vi "make arbitrary waveform_grMD.vi"() -> ()   [LabVIEW 2017]
doc: "SciScan 1.2 160622"
uses:
  Custom Controls/scan mode main settings tab.ctl
  Custom Controls/pixel resolution enum.ctl
  Custom Controls/experiment type.ctl
  GFG/GFGDisplayRefsGet.vi
  GFG/GFGnumericGet.vi
  GFG/GFGfpRefGet.vi
  GFG/GFGImageRefsGet.vi
  GFG/GFGpathGet.vi
  GFG/GFG library.lvlib
  <vilib>/vision/NI_Vision_Development_Module.lvlib
panel:
  out "error out 5":errorcluster
  out "error out 4":errorcluster
  out "XY voltages of the current framescan":dbl[][][](array[numeric])
  out "x.pixels refreshed?":bool
  out "xy.voltage.map refreshed?":bool
  out "Linescan voltages refreshed?":bool
  out "linescan.xy.waveform refreshed?":bool
  out "ROI refreshed?":bool
  out "Source VI":string
  out "error out 3":errorcluster
  out "error out 2":errorcluster
  out "error out":errorcluster
  out "XY map":cluster{"Y":dbl[], "Y":dbl[]}[](graph)
  out "Final linescan xy voltage plot":cluster{"Y":dbl[], "Y":dbl[]}[](graph)
  out "XY linescan pixel map":cluster{"Y":dbl[], "Y":dbl[]}[](graph)
  out "Linescan y voltages per scan point":dbl[](graph)
  out "Linescan x voltages per scan point":dbl[](graph)
  out "Linescan y waveform":waveform(dbl)(graph)
  out "Linescan x waveform":waveform(dbl)(graph)
  out "Number of pixels per period":i32
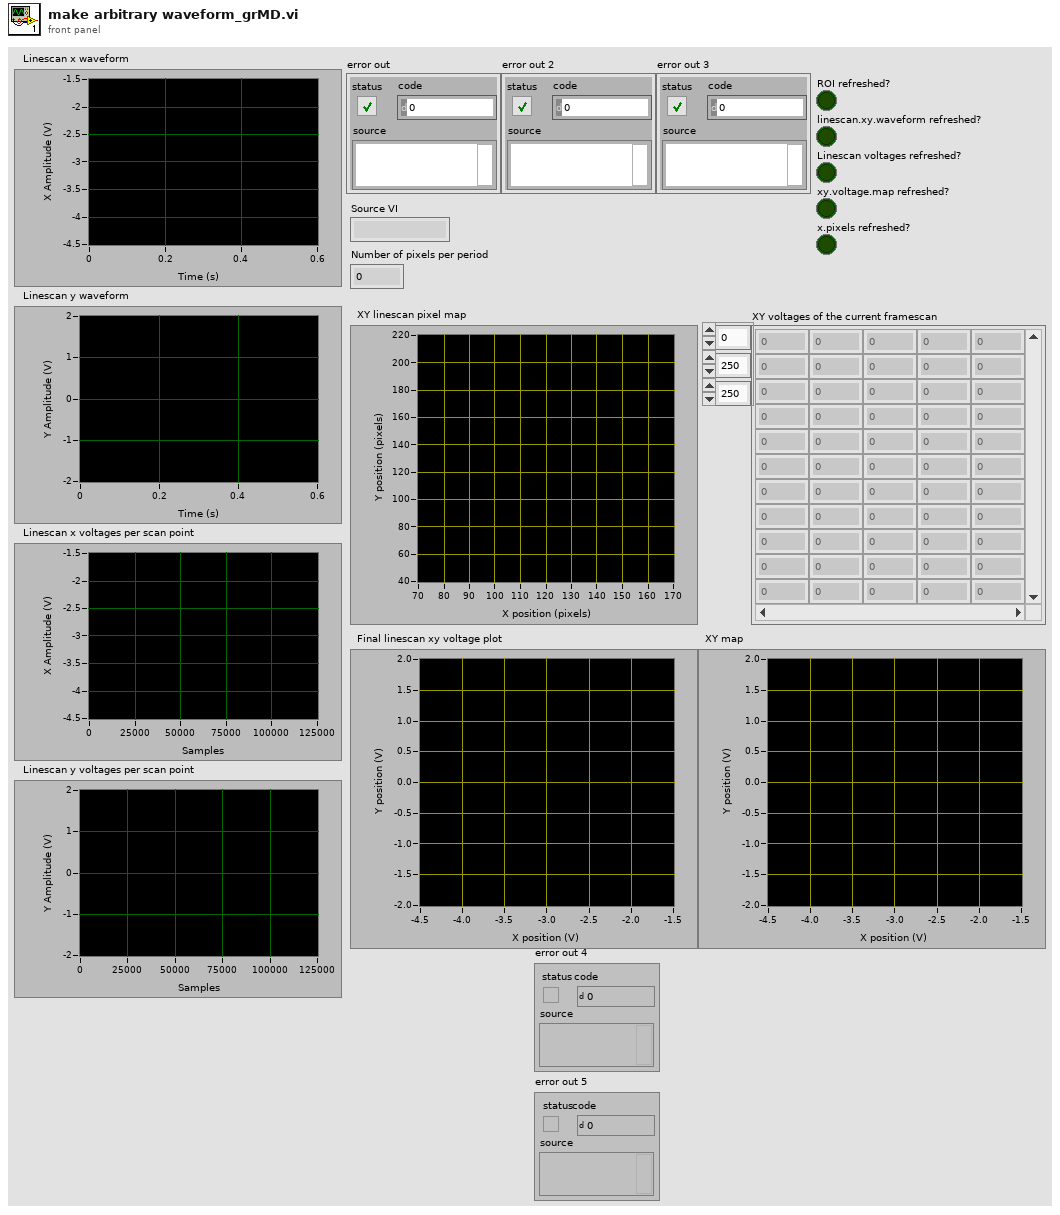
[diagram p1: front panel]
types:
  T1 = typedef "ROI Descriptor" = cluster{"Global Rectangle":i32[], "Contours":cluster{"ID":enum32{"External", "Internal"}, "Type":u32, "Coordinates":i32[]}[]}
  T2 = cluster{"Channel 1 small":refnum<vi>, "Channel 2 small":refnum<vi>, "Channel 3 small":refnum<vi>, "Channel 4 small":refnum<vi>, "Channel 1 large":refnum<vi>, "Channel 2 large":refnum<vi>, "Channel 3 large":refnum<vi>, "Channel 4 large":refnum<vi>, "RGB overlay":refnum<vi>, "ROI Image display":refnum<vi>, "arb line scan display":refnum<vi>, "Channel 5 large":refnum<vi>}
  T3 = cluster{"Global Rectangle":i32[], "Contours":cluster{"Contour Type":u32, "ROI Type":u32, "Points":i32[]}[]}
  T4 = cluster{"xyvoltagefor2frames":dbl[][][], "x.pixels":dbl, "nomin.x.pixels":dbl, "y.pixels":dbl, "fill.fraction":dbl, "x.bidirectional":bool, "y.bidirectional":bool}
  T5 = enum32{"Page Enabled", "Page Disabled", "Page Disabled & Grayed"}
  T6 = typedef "pixel resolution enum.ctl" = enum16{"128 x 128", "256 x 128", "256 x 256", "512 x  64", "512 x 128", "512 x 256", "512 x 512", "1024 x 512", "1024 x 1024", "arbitrary"}
  T7 = typedef "experiment type.ctl" = string
  T8 = enum8{"Enabled", "Disabled", "Disabled and Grayed Out"}
  T9 = typedef "scan mode main settings tab.ctl" = enum32{"2D frame", "2D line scan", "general settings", "Z Stack", "piezo"}
  T10 = cluster{"WaveformChartRef":refnum<vi>, "DigitalRef":refnum<vi>, "ArrayRef":refnum<vi>, "TabControlRef":refnum<vi>, "EnumRef":refnum<vi>, "RingRef":refnum<vi>, "BooleanRef":refnum<vi>, "KnobRef":refnum<vi>, "SlideRef":refnum<vi>, "PathRef":refnum<vi>, "StringRef":refnum<vi>, "ComboBox":refnum<vi>, "WaveformGraphRef":refnum<vi>}
  T11 = typedef "IMAQ Image.ctl" = refnum<image>
  T12 = cluster{"Channel 1 small":T11, "Channel 2 small":T11, "Channel 3 small":T11, "Channel 4 small":T11, "Channel 1 large":T11, "Channel 2 large":T11, "Channel 3 large":T11, "Channel 4 large":T11, "RGB overlay":T11, "ROI Image display":T11, "arb line scan display":T11, "Channel 5 large":T11}
  T13 = cluster{"ID":enum32{"External", "Internal"}, "Type":u32, "Coordinates":i32[]}[]
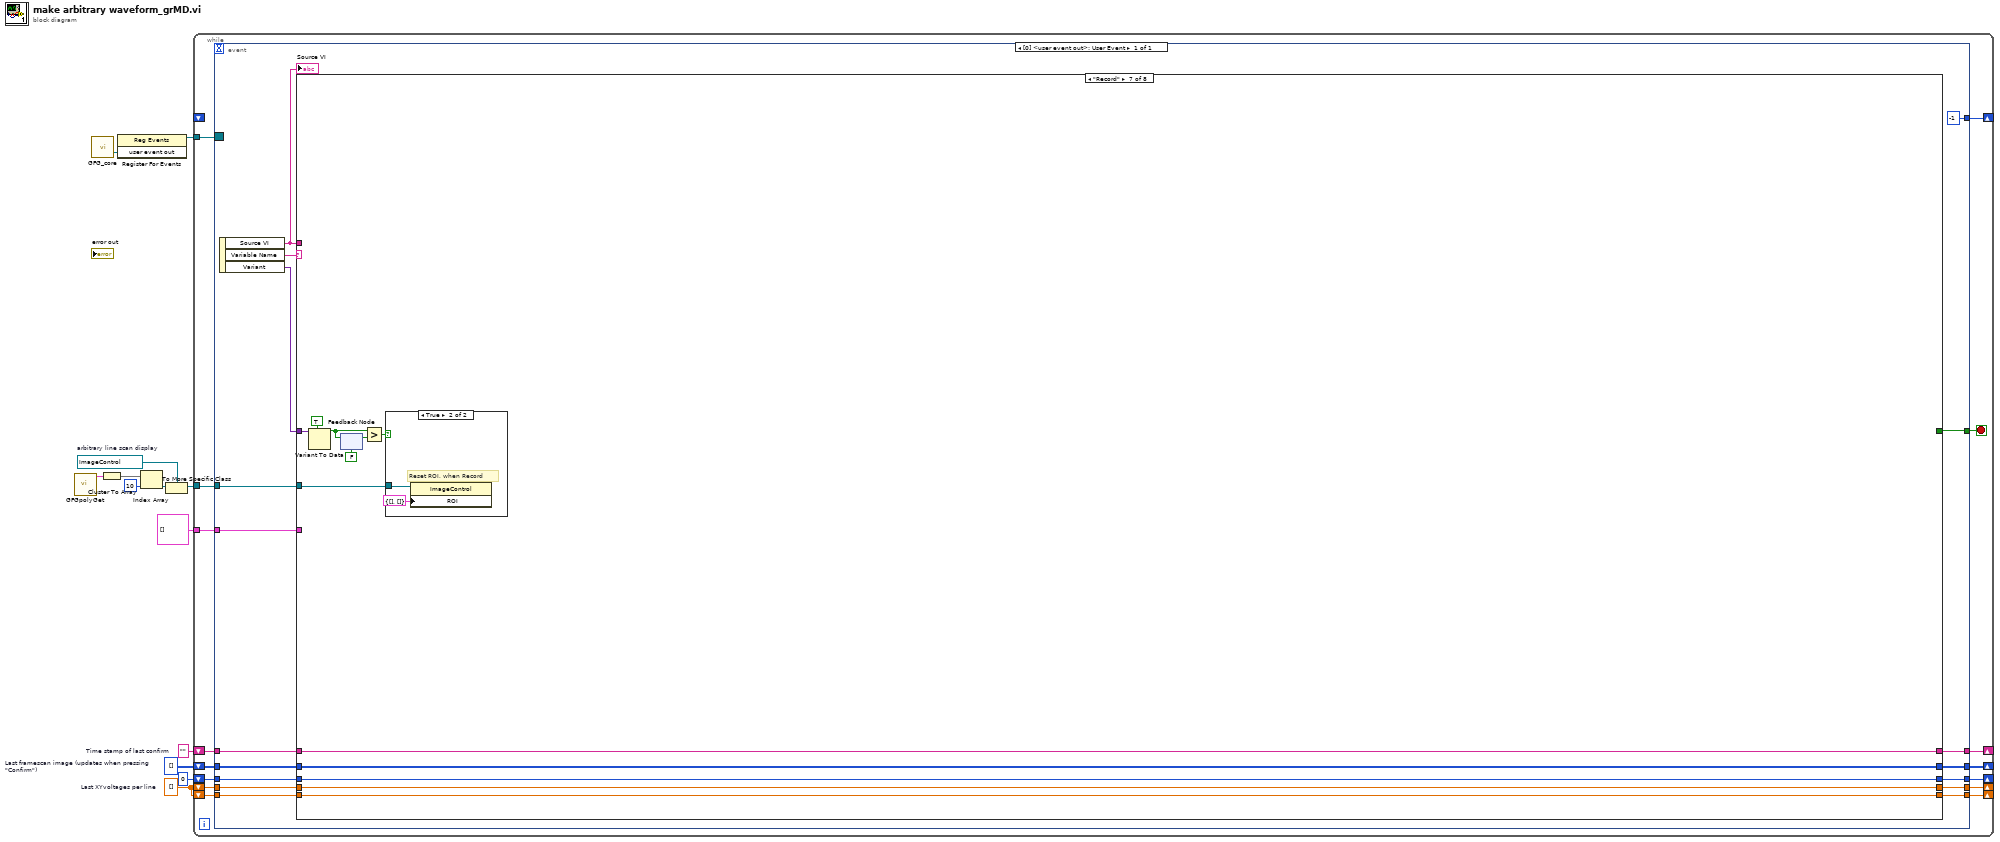
[diagram p0: block diagram]
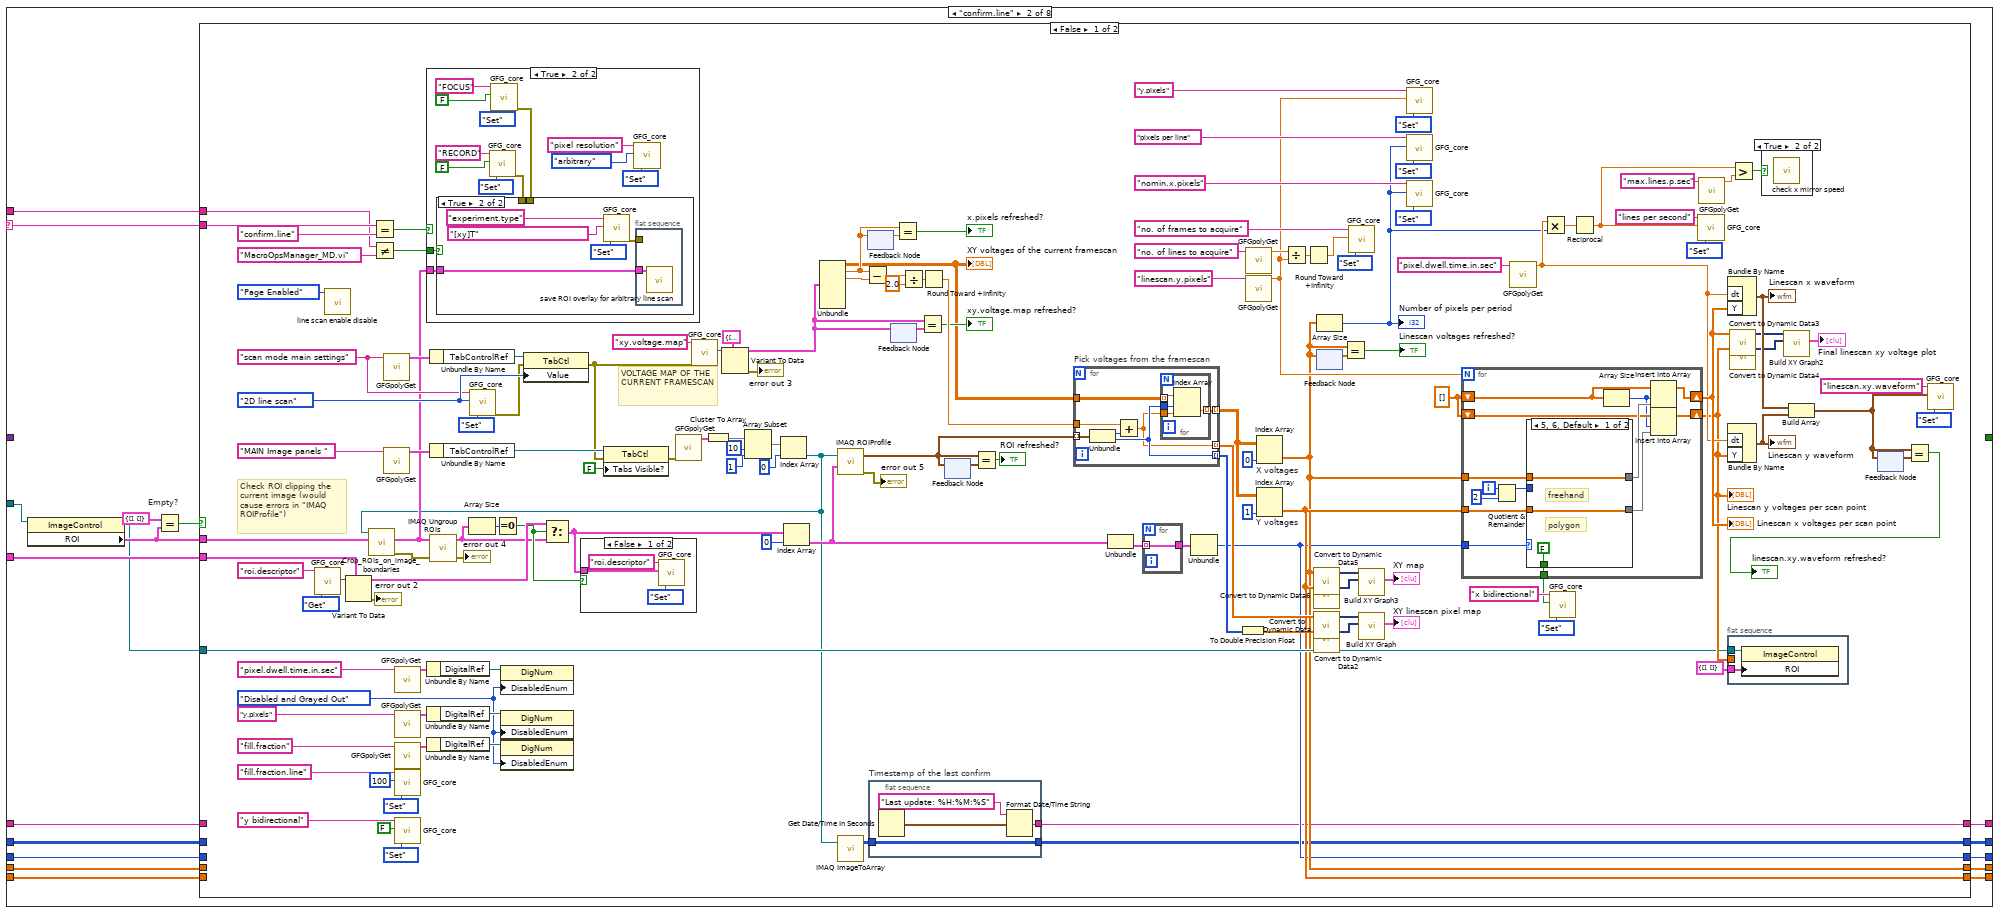
[diagram p3: hidden frame]
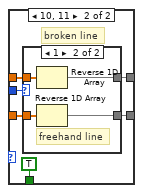
[diagram p8: hidden frame]
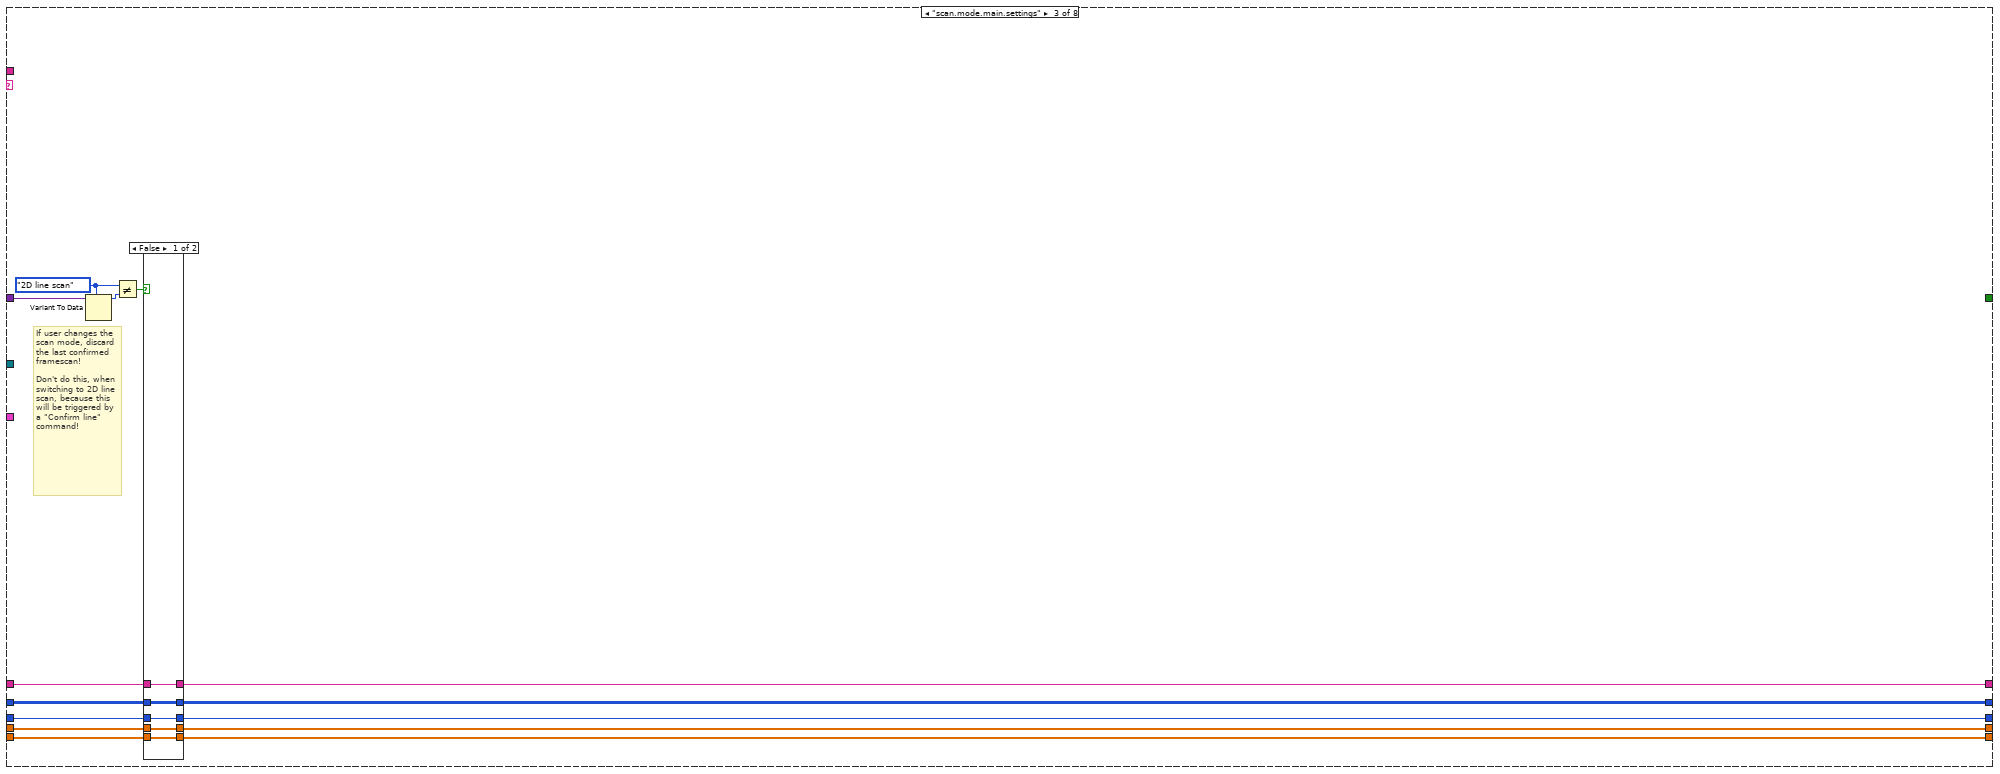
[diagram p11: hidden frame]
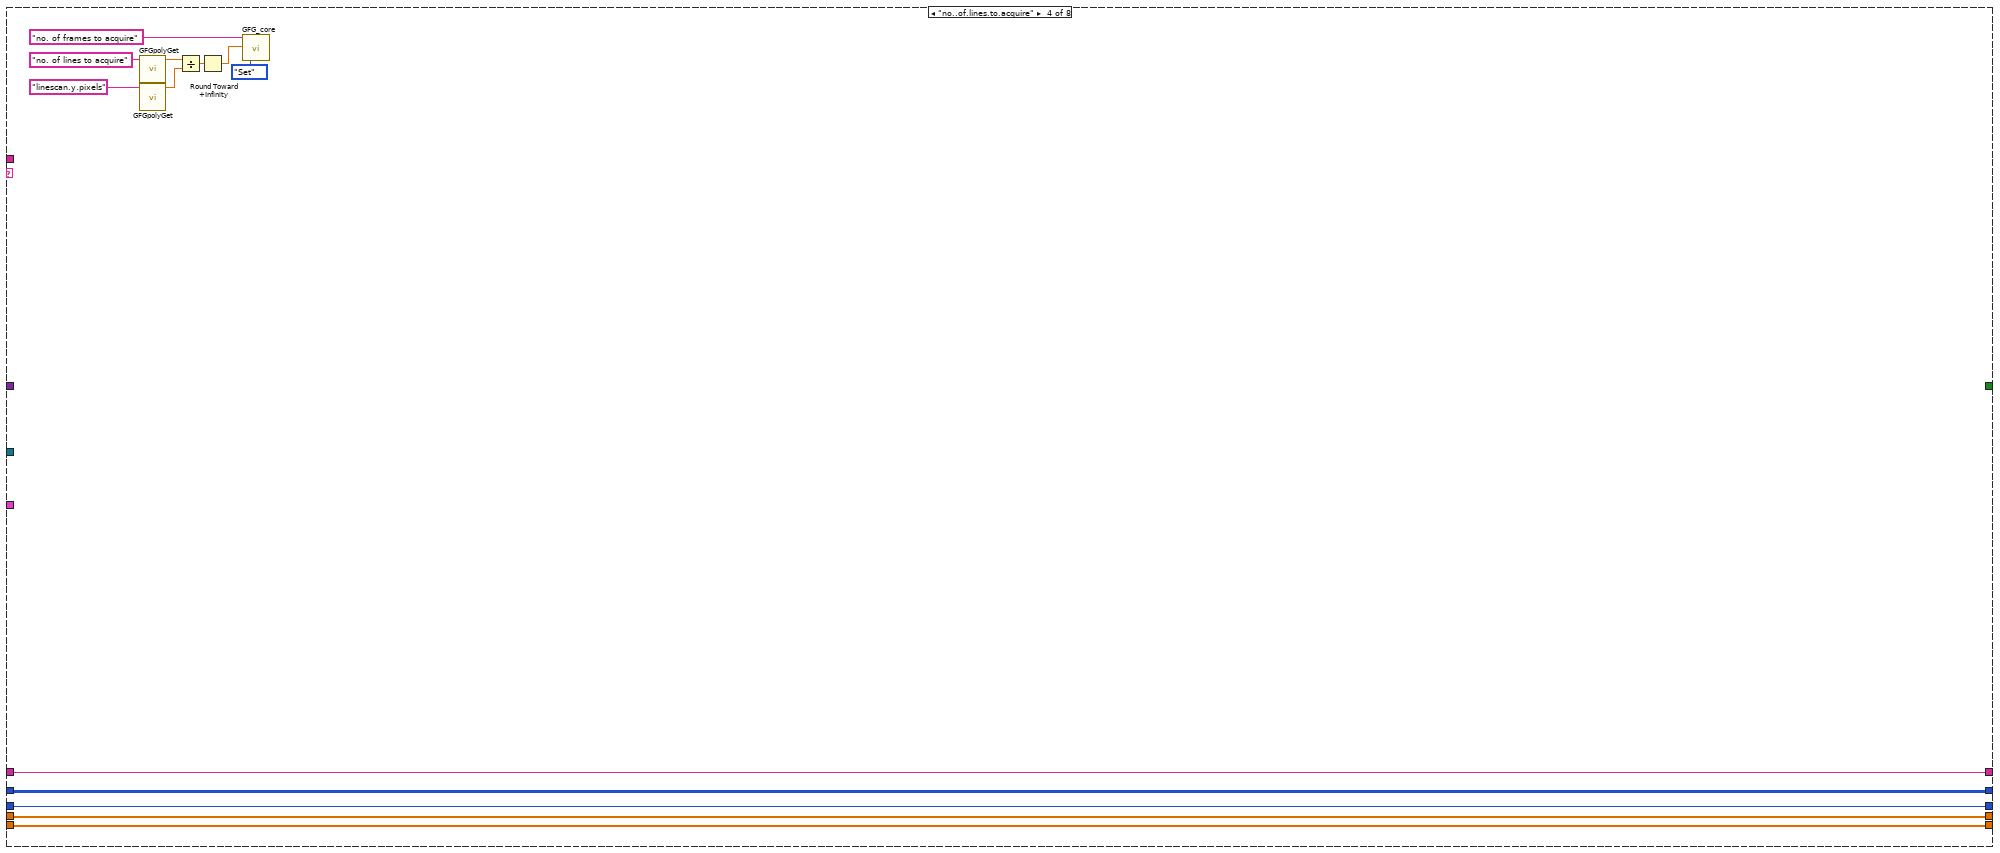
[diagram p13: hidden frame]
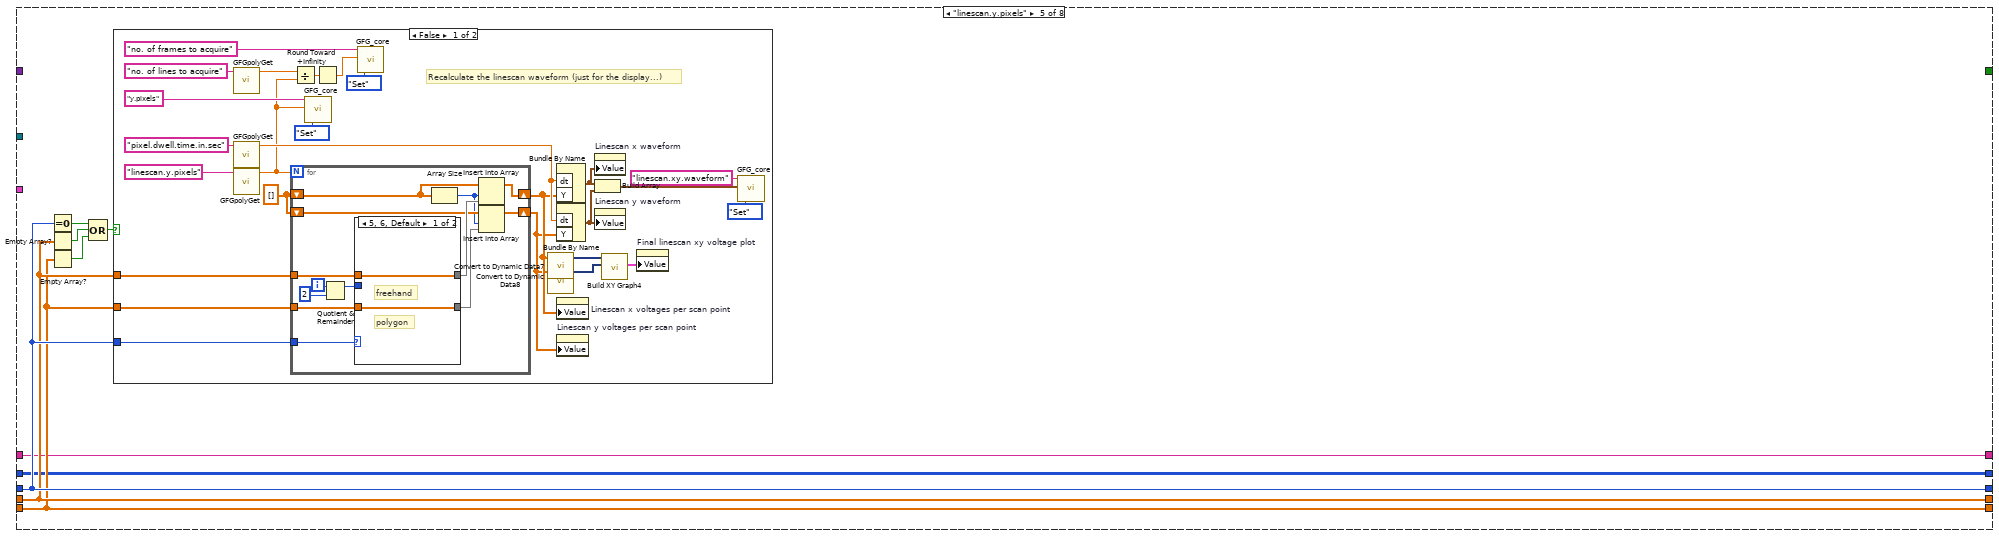
[diagram p14: hidden frame]
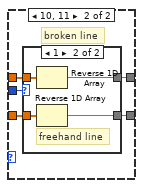
[diagram p15: hidden frame]
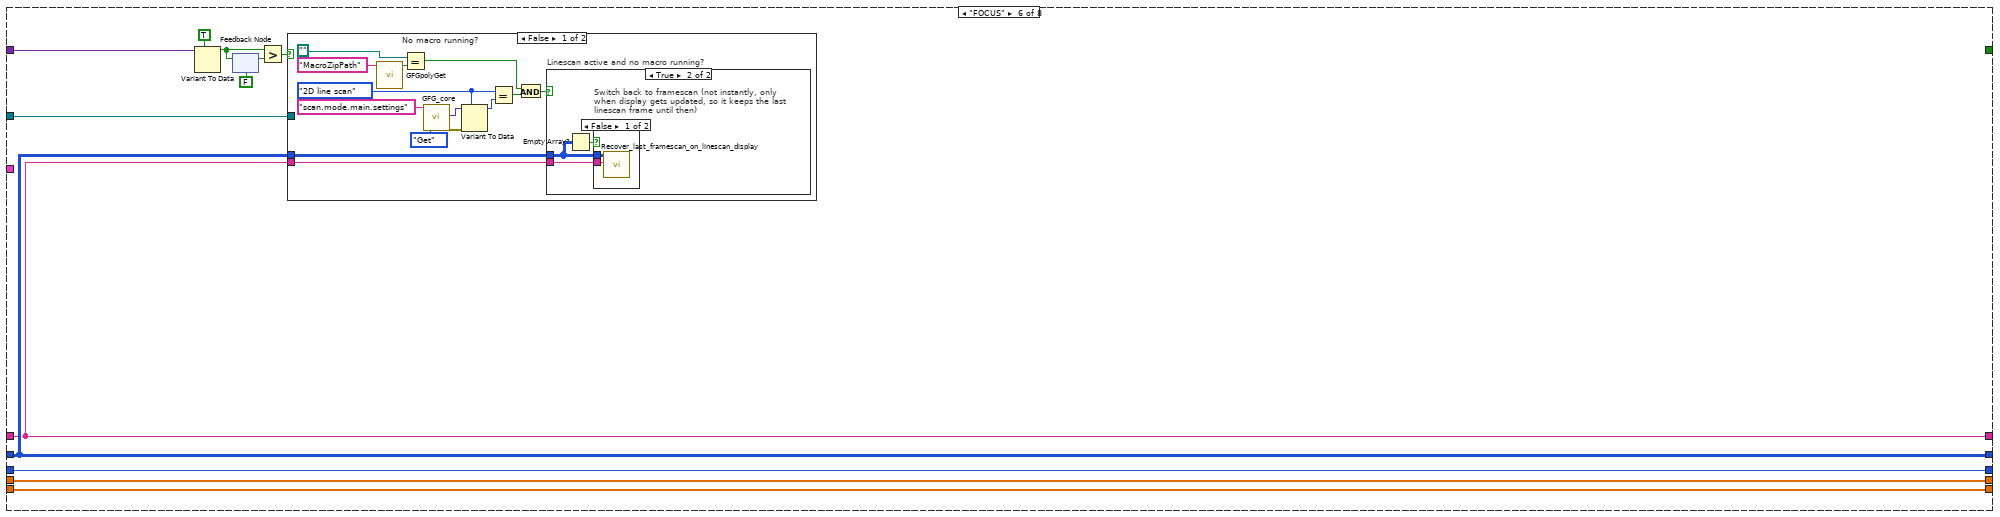
[diagram p18: hidden frame]
diagram:
  w1 = ""  # Time stamp of last confirm
  w2 = i16[][] []  # Last framescan image (updates when pressing "Confirm")
  w3 = dbl[] []  # Last XYvoltages per line
  w11 = refnum<vi> refnum  # arbitrary line scan display
  n1 = call-poly "GFGpolyGet.vi"() -> ("DisplayRefsOut(generic class)"=w10:T2)  [unwired: 10 in, 1 out]
  n2 = call "GFG_core.vi"() -> ("user event out"=w12:refnum<user-event>)  [unwired: 13 in, 6 out]
  n3 = Cluster To Array(cluster=w10) -> (array=w8:refnum<vi>[])
  n4 = register-events(w12) -> (reference out=w13:refnum<event-registration>)  [unwired: 2 in, 1 out]
  n5 = Index Array(array=w8, index=10) -> (element=w6:refnum<vi>)
  n6 = To More Specific Class(target class=w11, reference=w6) -> (specific class reference=w9:refnum<vi>)  [unwired: 1 in, 1 out]
  n7 = while {
    tunnel: w13 -> [w28]
    shift-right: [w26] -> _
    shift-left: _ -> [_]
    tunnel: w9 -> [w25]
    tunnel: T1[] [] ("ROI Descriptors out") -> [w24]
    shift-right: [w22] -> _
    shift-left: w3 -> [w20]
    shift-right: [w23] -> _
    shift-left: w3 -> [w19]
    shift-right: [w21] -> _
    shift-left: u32 0 ("Type") -> [w18]
    shift-right: [w17] -> _
    shift-left: w2 -> [w16]
    shift-right: [w15] -> _
    shift-left: w1 -> [w14]
    stop <- w27 stop-if-true
    n8 = event shown="[0] <user event out>: User Event" {
      selector: w28 -> [_]
      dyn-events: _ -> [_]
      timeout: _ -> [_]
      tunnel: w25 -> [w45]
      tunnel: [w42] -> w27
      tunnel: [-1 ("length")] -> w26
      tunnel: w24 -> [w39]
      tunnel: [w38] -> w23
      tunnel: [w37] -> w22
      tunnel: [w36] -> w21
      tunnel: w20 -> [w35]
      tunnel: w19 -> [w34]
      tunnel: w18 -> [w33]
      tunnel: [w32] -> w17
      tunnel: w16 -> [w31]
      tunnel: [w30] -> w15
      tunnel: w14 -> [w29]
      event User Event {
        n9 = event-data() -> ("Source VI"=w41:string, "Variable Name"=w43:string, "Variant"=w40:variant)  [unwired: 1 in]
        "Source VI" <- w41
        n10 = case shown="\"Record\"" w43 {
          selector: w43 -> [_ w63 _ _ _ _ _ _]
          tunnel: w45 -> [_ w68 _ _ _ w380 w422 _]
          tunnel: w40 -> [_ _ w298 _ _ w389 w423 w437]
          tunnel: [_ _ _ _ _ _ _ w436] -> w42
          tunnel: w41 -> [_ w67 _ _ _ _ _ _]
          tunnel: w39 -> [_ w66 _ _ _ _ _ _]
          tunnel: [w50 w61 w285 w306 w323 w386 w419 w435] -> w38
          tunnel: [w49 w60 w286 w307 w324 w387 w420 w434] -> w37
          tunnel: [w48 w59 w287 w308 w325 w388 w421 w433] -> w36
          tunnel: w35 -> [w49 w57 w291 w307 w324 w387 w420 w434]
          tunnel: w34 -> [w50 w56 w290 w306 w323 w386 w419 w435]
          tunnel: w33 -> [w48 w58 w292 w308 w325 w388 w421 w433]
          tunnel: [w47 w54 w288 w305 w318 w379 w418 w432] -> w32
          tunnel: w31 -> [w47 w53 w293 w305 w318 w379 w418 w432]
          tunnel: [w46 w52 w289 w304 w317 w378 w417 w431] -> w30
          tunnel: w29 -> [w46 w51 w294 w304 w317 w378 w417 w431]
          frame Default {
          }
          frame "confirm.line" {
            n11 = property class="ImageControl"(reference=w68) -> (reference out=w55:refnum<vi>, "ROI"=w65:T3)  [unwired: 1 in, 1 out]
            n12 = Equal? "Empty?"(x=T3 {"Global Rectangle"=[], "Contours"=[]} ("ROI"), y=w65) -> (x = y?=w62:bool)
            n13 = case shown="False" w62 {
              tunnel: w55 -> [w158 _]
              tunnel: w63 -> [w121 _]
              tunnel: w67 -> [w93 _]
              tunnel: w66 -> [w87 _]
              tunnel: w65 -> [w74 _]
              tunnel: [w81 w282] -> w61
              tunnel: [w80 w283] -> w60
              tunnel: [w79 w284] -> w59
              tunnel: w58 -> [_ w284]
              tunnel: w57 -> [_ w283]
              tunnel: w56 -> [_ w282]
              tunnel: [w76 w281] -> w54
              tunnel: w53 -> [_ w281]
              tunnel: [w75 w280] -> w52
              tunnel: w51 -> [_ w280]
              frame False {
                w86 = T8."Disabled and Grayed Out" ("Disabled")
                w90 = scan_mode_main_settings_tab."2D line scan" ("scan mode main settings")
                w89 = "scan mode main settings" ("Variable Name in")
                w195 = dbl[] []
                # "Check ROI clipping the current image (would cause errors in \"IMAQ ROIProfile\")"
                # "VOLTAGE MAP OF THE CURRENT FRAMESCAN"
                n14 = call "GFG_core.vi"("Variable Name in"="roi.descriptor", "Action"=enum16{"Init", "Set", "Get"}."Get") -> ("Variant Out"=w153:variant)  [unwired: 11 in, 6 out]
                n15 = call "line scan enable disable.vi"("Page Enabled State"=T5."Page Enabled") -> ()  [unwired: 11 in]
                n16 = Variant To Data(type=w87, Variant=w153) -> (data=w117:T1[], error out=→"error out 2":errorcluster)  [unwired: 1 in]
                n17 = Equal?(x=w121, y="confirm.line") -> (x = y?=w119:bool)
                n18 = Not Equal?(x=w93, y="MacroOpsManager_MD.vi") -> (x != y?=w92:bool)
                n19 = call-poly "GFGpolyGet.vi"("Variable Name in"=w89) -> ("output cluster"=w171:T10)  [unwired: 9 in, 1 out]
                n20 = call-poly "GFGpolyGet.vi"("Variable Name in"="MAIN Image panels ") -> ("output cluster"=w175:T10)  [unwired: 9 in, 1 out]
                n21 = call-poly "GFGpolyGet.vi"("Variable Name in"="pixel.dwell.time.in.sec") -> ("output cluster"=w162:T10)  [unwired: 9 in, 1 out]
                n22 = call-poly "GFGpolyGet.vi"("Variable Name in"="y.pixels") -> ("output cluster"=w123:T10)  [unwired: 9 in, 1 out]
                n23 = call-poly "GFGpolyGet.vi"("Variable Name in"="fill.fraction") -> ("output cluster"=w128:T10)  [unwired: 9 in, 1 out]
                n24 = call "GFG_core.vi"("Variable Name in"="fill.fraction.line", "Variant in"=100 ("y"), "Action"=enum16{"Init", "Set", "Get"}."Set") -> ()  [unwired: 10 in, 7 out]
                n25 = call "GFG_core.vi"("Variable Name in"="y bidirectional", "Variant in"=FALSE, "Action"=enum16{"Init", "Set", "Get"}."Set") -> ()  [unwired: 10 in, 7 out]
                n26 = Unbundle By Name(w162) -> ("DigitalRef"=w163:refnum<vi>)
                n27 = Unbundle By Name(w123) -> ("DigitalRef"=w122:refnum<vi>)
                n28 = Unbundle By Name(w128) -> ("DigitalRef"=w129:refnum<vi>)
                n29 = Unbundle By Name(w171) -> ("TabControlRef"=w172:refnum<vi>)
                n30 = Unbundle By Name(w175) -> ("TabControlRef"=w173:refnum<vi>)
                n31 = call "GFG_core.vi"("Variable Name in"=w89, "Variant in"=w90, "Action"=enum16{"Init", "Set", "Get", "Clear"}."Set") -> ("error out"=w88:errorcluster)  [unwired: 10 in, 6 out]
                n32 = property class="DigNum"(reference=w163, "DisabledEnum"=w86) -> ()  [unwired: 1 in, 2 out]
                n33 = property class="DigNum"(reference=w122, "DisabledEnum"=w86) -> ()  [unwired: 1 in, 2 out]
                n34 = property class="DigNum"(reference=w129, "DisabledEnum"=w86) -> ()  [unwired: 1 in, 2 out]
                n35 = property class="TabCtl"(reference=w172, error in=w88, "Value"=w90) -> (error out=w97:errorcluster)  [unwired: 1 out]
                n36 = property class="TabCtl"(reference=w173, error in=w97, "Tabs Visible?"=FALSE) -> (error out=w96:errorcluster)  [unwired: 1 out]
                n37 = call-poly "GFGpolyGet.vi"("error in (no error)"=w96) -> ("Image Refs Out"=w209:T12)  [unwired: 9 in, 1 out]
                n38 = call "GFG_core.vi"("Variable Name in"="xy.voltage.map", "error in (no error)"=w97) -> ("Variant Out"=w200:variant)  [unwired: 11 in, 6 out]
                n39 = Cluster To Array(cluster=w209) -> (array=w208:T11[])
                n40 = Variant To Data(type=T4 {"xyvoltagefor2frames"=[], "x.pixels"=0.0, "nomin.x.pixels"=0.0, "y.pixels"=0.0, "fill.fraction"=0.0, "x.bidirectional"=FALSE, "y.bidirectional"=FALSE} ("output cluster"), Variant=w200) -> (data=w100:T4, error out=→"error out 3":errorcluster)  [unwired: 1 in]
                n41 = Array Subset(array=w208, index=10, length=1) -> (w204:T11[])
                n42 = Index Array(array=w204, index=0) -> (element=w71:T11)
                n43 = call "Crop_ROIs_on_image_boundaries.vi"("ROI Descriptor IN"=w74, "Image"=w71) -> ("error out"=w70:errorcluster, "ROI Descriptor OUT"=w73:T1)  [unwired: 8 in]
                n44 = case shown="True" w119 {
                  tunnel: w73 -> [_ w225]
                  tunnel: w92 -> [_ w224]
                  frame False {
                  }
                  frame True {
                    n45 = call "GFG_core.vi"("Variable Name in"="RECORD", "Variant in"=FALSE, "Action"=enum16{"Init", "Set", "Get"}."Set") -> ("error out"=w222:errorcluster)  [unwired: 10 in, 6 out]
                    n46 = call "GFG_core.vi"("Variable Name in"="FOCUS", "Variant in"=FALSE, "Action"=enum16{"Init", "Set", "Get"}."Set") -> ("error out"=w223:errorcluster)  [unwired: 10 in, 6 out]
                    n47 = case shown="True" w224 {
                      tunnel: w225 -> [_ w235]
                      tunnel: w223 -> [_ _]
                      tunnel: w222 -> [_ _]
                      frame False {
                      }
                      frame True {
                        n48 = call "GFG_core.vi"("Variable Name in"="experiment.type", "Variant in"=T7 "[xy]T" ("experiment type"), "Action"=enum16{"Init", "Set", "Get"}."Set") -> ("error out"=w232:errorcluster)  [unwired: 10 in, 6 out]
                        n49 = flat-sequence {
                          tunnel: w235 -> [w236]
                          tunnel: w232 -> [_]
                          frame #0 {
                            n50 = call "save ROI overlay for arbitrary line scan.vi"("ROI Descriptor"=w236) -> ()  [unwired: 11 in]
                          }
                        }
                      }
                    }
                    n51 = call "GFG_core.vi"("Variable Name in"="pixel resolution", "Variant in"=pixel_resolution_enum."arbitrary" ("pixel resolution"), "Action"=enum16{"Init", "Set", "Get"}."Set") -> ()  [unwired: 10 in, 7 out]
                  }
                }
                n52 = call "IMAQ Ungroup ROIs"("error in (no error)"=w70, "ROI Descriptor"=w73) -> ("error out"=→"error out 4":errorcluster, "ROI Descriptors out"=w95:T1[])  [unwired: 2 in]
                n53 = Array Size(array=w95) -> (size(s)=w154:i32)
                n54 = Equal To 0?(x=w154) -> (x = 0?=w115:bool)
                n55 = Select(t=w117, s=w115, f=w95) -> (s? t:f=w114:T1[])
                n56 = case shown="False" w115 {
                  tunnel: w114 -> [w215 _]
                  frame False {
                    n57 = call "GFG_core.vi"("Variable Name in"="roi.descriptor", "Variant in"=w215, "Action"=enum16{"Init", "Set", "Get"}."Set") -> ()  [unwired: 10 in, 7 out]
                  }
                  frame True {
                  }
                }
                n58 = Index Array(array=w114, index=0) -> (element=w116:T1)
                n59 = Unbundle(w100) -> ("xyvoltagefor2frames"=w78:dbl[][][], "x.pixels"=w99:dbl, "nomin.x.pixels"=w98:dbl)  [unwired: 4 out]
                "XY voltages of the current framescan" <- w78
                n60 = call "IMAQ ROIProfile"("ROI Descriptor"=w116, "Image"=w71) -> ("error out"=→"error out 5":errorcluster, "Pixel Coordinates"=w113:cluster{"X":u32, "Y":u32}[])  [unwired: 2 in, 3 out]
                n61 = call "IMAQ ImageToArray"("Image"=w71) -> ("Image Pixels (I16)"=w77:i16[][])  [unwired: 3 in, 4 out]
                n62 = Subtract(x=w99, y=w98) -> (x-y=w147:dbl)
                n63 = feedback #1() -> (w103:dbl)  [unwired: 1 in]
                n64 = feedback-in #1(w99) -> ()
                n65 = flat-sequence "Timestamp of the last confirm" {
                  tunnel: w77 -> [w214]
                  tunnel: [w214] -> w76
                  tunnel: [w211] -> w75
                  frame #0 {
                    n66 = Get Date/Time In Seconds() -> (seconds since 1Jan1904=w213:timestamp)
                    n67 = Format Date/Time String(time format string (%c)="Last update: %H:%M:%S", seconds (now)=w213) -> (date/time string=w211:string)  [unwired: 1 in]
                  }
                }
                n68 = feedback #2() -> (w104:T4)  [unwired: 1 in]
                n69 = feedback-in #2(w100) -> ()
                n70 = Equal?(x=w99, y=w103) -> (x = y?=→"x.pixels refreshed?":bool)
                n71 = Divide(x=w147, y=2.0) -> (x/y=w145:dbl)
                n72 = Equal?(x=w100, y=w104) -> (x = y?=→"xy.voltage.map refreshed?":bool)
                n73 = Round Toward +Infinity(x=w145) -> (ceil(x): smallest int >= x=w144:dbl)
                n74 = feedback #3() -> (w112:cluster{"X":u32, "Y":u32}[])  [unwired: 1 in]
                n75 = feedback-in #3(w113) -> ()
                n76 = Equal?(x=w113, y=w112) -> (x = y?=→"ROI refreshed?":bool)
                n77 = for "Pick voltages from the framescan" {
                  tunnel: w113 -> [w274] mode=indexing
                  tunnel: [w272] -> w203 mode=indexing
                  tunnel: w78 -> [w273]
                  tunnel: [w271] -> w84 mode=indexing
                  tunnel: [w268] -> w202 mode=indexing
                  tunnel: w144 -> [w269]
                  n78 = Unbundle(w274) -> ("X"=w270:u32, "Y"=w271:u32)
                  n79 = Add(x=w269, y=w270) -> (x+y=w268:dbl)
                  n80 = for {
                    tunnel: w273 -> [w278] mode=indexing
                    tunnel: w268 -> [w277]
                    tunnel: w271 -> [w276]
                    tunnel: [w275] -> w272 mode=indexing
                    n81 = Index Array(array=w278, index (row)=w276, index (col)=w277) -> (element=w275:dbl)
                  }
                }
                n82 = Unbundle(w116) -> ("Contours"=w206:T13)  [unwired: 1 out]
                n83 = for {
                  tunnel: w206 -> [w279] mode=indexing
                  tunnel: [w279] -> w205
                }
                n84 = Unbundle(w205) -> ("Type"=w79:u32)  [unwired: 2 out]
                n85 = To Double Precision Float(number=w84) -> (double precision float=w83:dbl[])
                n86 = call-poly "GFGpolyGet.vi"("Variable Name in"="no. of lines to acquire") -> ("Numeric"=w137:dbl)  [unwired: 8 in, 2 out]
                n87 = call-poly "GFGpolyGet.vi"("Variable Name in"="linescan.y.pixels") -> ("Numeric"=w136:dbl)  [unwired: 8 in, 2 out]
                n88 = Index Array "X voltages"(array=w203, index (col)=0 ("disabled index (col)")) -> (element=w80:dbl[])  [unwired: 1 in]
                n89 = Index Array "Y voltages"(array=w203, index (col)=1 ("disabled index (col)")) -> (element=w81:dbl[])  [unwired: 1 in]
                n90 = Divide(x=w137, y=w136) -> (x/y=w135:dbl)
                n91 = Round Toward +Infinity(x=w135) -> (ceil(x): smallest int >= x=w134:dbl)
                n92 = call "Convert to Dynamic Data5"("Array"=w80) -> ("Dynamic Data Type"=w190:dynamicdata)  [unwired: 3 in]
                n93 = call "Convert to Dynamic Data6"("Array"=w81) -> ("Dynamic Data Type"=w191:dynamicdata)  [unwired: 3 in]
                n94 = call "Convert to Dynamic Data"("Array"=w202) -> ("Dynamic Data Type"=w193:dynamicdata)  [unwired: 3 in]
                n95 = call "Convert to Dynamic Data2"("Array"=w83) -> ("Dynamic Data Type"=w192:dynamicdata)  [unwired: 3 in]
                n96 = Array Size(array=w80) -> (size(s)=w141:i32)
                "Number of pixels per period" <- w141
                n97 = feedback #4() -> (w107:dbl[])  [unwired: 1 in]
                n98 = feedback-in #4(w80) -> ()
                n99 = Equal?(x=w80, y=w107) -> (x = y?=→"Linescan voltages refreshed?":bool)
                n100 = call "GFG_core.vi"("Variable Name in"="no. of frames to acquire", "Variant in"=w134, "Action"=enum16{"Init", "Set", "Get"}."Set") -> ()  [unwired: 10 in, 7 out]
                n101 = call "Build XY Graph3"("Y Input"=w191, "X Input"=w190) -> ("XY Graph"=→"XY map":cluster{"Y":dbl[], "Y":dbl[]}[])  [unwired: 3 in, 6 out]
                n102 = call "Build XY Graph"("Y Input"=w192, "X Input"=w193) -> ("XY Graph"=→"XY linescan pixel map":cluster{"Y":dbl[], "Y":dbl[]}[])  [unwired: 3 in, 6 out]
                n103 = call "GFG_core.vi"("Variable Name in"="y.pixels", "Variant in"=w136, "Action"=enum16{"Init", "Set", "Get"}."Set") -> ()  [unwired: 10 in, 7 out]
                n104 = call "GFG_core.vi"("Variable Name in"="pixels per line", "Variant in"=w141, "Action"=enum16{"Init", "Set", "Get"}."Set") -> ()  [unwired: 10 in, 7 out]
                n105 = call "GFG_core.vi"("Variable Name in"="nomin.x.pixels", "Variant in"=w141, "Action"=enum16{"Init", "Set", "Get"}."Set") -> ()  [unwired: 10 in, 7 out]
                n106 = for {
                  N: w136 -> [_]
                  tunnel: w81 -> [w250]
                  tunnel: w80 -> [w252]
                  tunnel: w79 -> [w251]
                  shift-right: [w246] -> w180
                  shift-left: w195 -> [w241]
                  shift-right: [w244] -> w159
                  shift-left: w195 -> [w242]
                  tunnel: [w239] -> w149
                  i -> [w249]
                  n107 = Quotient & Remainder(x=w249, y=2) -> (x-y*floor(x/y)=w247:i32)  [unwired: 1 out]
                  n108 = case shown="5, 6, Default" w251 {
                    tunnel: w250 -> [w253 w260]
                    tunnel: w252 -> [w254 w261]
                    tunnel: [w254 w259] -> w245
                    tunnel: [w253 w258] -> w243
                    tunnel: w247 -> [_ w257]
                    tunnel: [FALSE TRUE] -> w239
                    frame 5, 6, Default {
                      # "freehand"
                      # "polygon"
                    }
                    frame 10, 11 {
                      # "broken line"
                      n109 = case shown="1" w257 {
                        tunnel: w261 -> [w263 w267]
                        tunnel: w260 -> [w262 w266]
                        tunnel: [w263 w265] -> w259
                        tunnel: [w262 w264] -> w258
                        frame 0, Default {
                        }
                        frame 1 {
                          # "freehand line"
                          n110 = Reverse 1D Array(array=w267) -> (reversed array=w265:dbl[])
                          n111 = Reverse 1D Array(array=w266) -> (reversed array=w264:dbl[])
                        }
                      }
                    }
                  }
                  n112 = Array Size(array=w241) -> (size(s)=w240:i32)
                  n113 = Insert Into Array(array=w241, index=w240, new element=w245) -> (w246:dbl[])
                  n114 = Insert Into Array(array=w242, index=w240, new element=w243) -> (w244:dbl[])
                }
                "Linescan x voltages per scan point" <- w180
                "Linescan y voltages per scan point" <- w159
                n115 = call-poly "GFGpolyGet.vi"("Variable Name in"="pixel.dwell.time.in.sec" ("Tag in")) -> ("Numeric"=w166:dbl)  [unwired: 8 in, 2 out]
                n116 = Multiply(x=w166, y=w141) -> (x*y=w165:dbl)
                n117 = call "GFG_core.vi"("Variable Name in"="x bidirectional", "Variant in"=w149, "Action"=enum16{"Init", "Set", "Get"}."Set") -> ()  [unwired: 10 in, 7 out]
                n118 = Reciprocal(x=w165) -> (1/x=w133:dbl)
                n119 = call "GFG_core.vi"("Variable Name in"="lines per second", "Variant in"=w133, "Action"=enum16{"Init", "Set", "Get"}."Set") -> ()  [unwired: 10 in, 7 out]
                n120 = call-poly "GFGpolyGet.vi"("Variable Name in"="max.lines.p.sec") -> ("Numeric"=w131:dbl)  [unwired: 8 in, 2 out]
                n121 = Bundle By Name("dt"=w166, "Y"=w180) -> (w182:waveform(dbl))  [unwired: 1 in]
                "Linescan x waveform" <- w182
                n122 = Bundle By Name("dt"=w166, "Y"=w159) -> (w183:waveform(dbl))  [unwired: 1 in]
                "Linescan y waveform" <- w183
                n123 = flat-sequence {
                  tunnel: w159 -> [_]
                  tunnel: w158 -> [w237]
                  tunnel: T3 {"Global Rectangle"=[], "Contours"=[]} ("ROI") -> [w238]
                  frame #0 {
                    n124 = property class="ImageControl"(reference=w237, "ROI"=w238) -> ()  [unwired: 1 in, 2 out]
                  }
                }
                n125 = call "Convert to Dynamic Data3"("Array"=w180) -> ("Dynamic Data Type"=w179:dynamicdata)  [unwired: 3 in]
                n126 = call "Convert to Dynamic Data4"("Array"=w159) -> ("Dynamic Data Type"=w178:dynamicdata)  [unwired: 3 in]
                n127 = Greater?(x=w133, y=w131) -> (0:w130:bool)
                n128 = case shown="True" w130 {
                  frame False {
                  }
                  frame True {
                    n129 = call "check x mirror speed.vi"() -> ()  [unwired: 11 in, 1 out]
                  }
                }
                n130 = call "Build XY Graph2"("Y Input"=w178, "X Input"=w179) -> ("XY Graph"=→"Final linescan xy voltage plot":cluster{"Y":dbl[], "Y":dbl[]}[])  [unwired: 3 in, 6 out]
                n131 = Build Array(w182, w183) -> (w108:waveform(dbl)[])
                n132 = feedback #5() -> (w109:waveform(dbl)[])  [unwired: 1 in]
                n133 = feedback-in #5(w108) -> ()
                n134 = Equal?(x=w108, y=w109) -> (x = y?=→"linescan.xy.waveform refreshed?":bool)
                n135 = call "GFG_core.vi"("Variable Name in"="linescan.xy.waveform", "Variant in"=w108, "Action"=enum16{"Init", "Set", "Get"}."Set") -> ()  [unwired: 10 in, 7 out]
              }
              frame True {
                # "Don't do anything, when there is no ROI selected!"
              }
            }
          }
          frame "scan.mode.main.settings" {
            w296 = scan_mode_main_settings_tab."2D line scan" ("scan mode main settings")
            # "If user changes the scan mode, discard the last confirmed framescan!\n\nDon't do this, when switching to 2D line scan, because this will be triggered by a \"Confirm line\" command!"
            n136 = Variant To Data(type=w296, Variant=w298) -> (data=w297:T9)  [unwired: 1 in, 1 out]
            n137 = Not Equal?(x=w296, y=w297) -> (x != y?=w295:bool)
            n138 = case shown="False" w295 {
              tunnel: w294 -> [w303 _]
              tunnel: w293 -> [w302 _]
              tunnel: w292 -> [w301 _]
              tunnel: w291 -> [w300 _]
              tunnel: w290 -> [w299 _]
              tunnel: [w303 _] -> w289
              tunnel: [w302 _] -> w288
              tunnel: [w301 _] -> w287
              tunnel: [w300 _] -> w286
              tunnel: [w299 _] -> w285
              frame False {
              }
              frame True {
              }
            }
          }
          frame "no..of.lines.to.acquire" {
            n139 = call-poly "GFGpolyGet.vi"("Variable Name in"="no. of lines to acquire") -> ("Numeric"=w313:dbl)  [unwired: 8 in, 2 out]
            n140 = call-poly "GFGpolyGet.vi"("Variable Name in"="linescan.y.pixels") -> ("Numeric"=w312:dbl)  [unwired: 8 in, 2 out]
            n141 = Divide(x=w313, y=w312) -> (x/y=w311:dbl)
            n142 = Round Toward +Infinity(x=w311) -> (ceil(x): smallest int >= x=w310:dbl)
            n143 = call "GFG_core.vi"("Variable Name in"="no. of frames to acquire", "Variant in"=w310, "Action"=enum16{"Init", "Set", "Get"}."Set") -> ()  [unwired: 10 in, 7 out]
          }
          frame "linescan.y.pixels" {
            n144 = Equal To 0?(x=w325) -> (x = 0?=w322:bool)
            n145 = Empty Array?(array=w324) -> (empty?=w321:bool)
            n146 = Empty Array?(array=w323) -> (empty?=w320:bool)
            n147 = Compound Arithmetic op=OR(w322, w321, w320) -> (w319:bool)
            n148 = case shown="False" w319 {
              tunnel: w325 -> [w347 _]
              tunnel: w324 -> [w346 _]
              tunnel: w323 -> [w345 _]
              frame False {
                w348 = dbl[] []
                # "Recalculate the linescan waveform (just for the display...)"
                n149 = call-poly "GFGpolyGet.vi"("Variable Name in"="no. of lines to acquire") -> ("Numeric"=w330:dbl)  [unwired: 8 in, 2 out]
                n150 = call-poly "GFGpolyGet.vi"("Variable Name in"="pixel.dwell.time.in.sec" ("Tag in")) -> ("Numeric"=w343:dbl)  [unwired: 8 in, 2 out]
                n151 = call-poly "GFGpolyGet.vi"("Variable Name in"="linescan.y.pixels") -> ("Numeric"=w326:dbl)  [unwired: 8 in, 2 out]
                n152 = for {
                  N: w326 -> [_]
                  tunnel: w345 -> [w362]
                  tunnel: w346 -> [w364]
                  tunnel: w347 -> [w363]
                  shift-right: [w358] -> w336
                  shift-left: w348 -> [w353]
                  shift-right: [w356] -> w335
                  shift-left: w348 -> [w354]
                  i -> [w361]
                  n153 = Quotient & Remainder(x=w361, y=2) -> (x-y*floor(x/y)=w359:i32)  [unwired: 1 out]
                  n154 = case shown="5, 6, Default" w363 {
                    tunnel: w362 -> [w365 w370]
                    tunnel: w364 -> [w366 w371]
                    tunnel: [w366 w369] -> w357
                    tunnel: [w365 w368] -> w355
                    tunnel: w359 -> [_ w367]
                    frame 5, 6, Default {
                      # "freehand"
                      # "polygon"
                    }
                    frame 10, 11 {
                      # "broken line"
                      n155 = case shown="1" w367 {
                        tunnel: w371 -> [w373 w377]
                        tunnel: w370 -> [w372 w376]
                        tunnel: [w373 w375] -> w369
                        tunnel: [w372 w374] -> w368
                        frame 0, Default {
                        }
                        frame 1 {
                          # "freehand line"
                          n156 = Reverse 1D Array(array=w377) -> (reversed array=w375:dbl[])
                          n157 = Reverse 1D Array(array=w376) -> (reversed array=w374:dbl[])
                        }
                      }
                    }
                  }
                  n158 = Array Size(array=w353) -> (size(s)=w352:i32)
                  n159 = Insert Into Array(array=w353, index=w352, new element=w357) -> (w358:dbl[])
                  n160 = Insert Into Array(array=w354, index=w352, new element=w355) -> (w356:dbl[])
                }
                n161 = Divide(x=w330, y=w326) -> (x/y=w331:dbl)
                n162 = call "GFG_core.vi"("Variable Name in"="y.pixels", "Variant in"=w326, "Action"=enum16{"Init", "Set", "Get"}."Set") -> ()  [unwired: 10 in, 7 out]
                n163 = Round Toward +Infinity(x=w331) -> (ceil(x): smallest int >= x=w332:dbl)
                n164 = call "GFG_core.vi"("Variable Name in"="no. of frames to acquire", "Variant in"=w332, "Action"=enum16{"Init", "Set", "Get"}."Set") -> ()  [unwired: 10 in, 7 out]
                n165 = call "Convert to Dynamic Data7"("Array"=w336) -> ("Dynamic Data Type"=w338:dynamicdata)  [unwired: 3 in]
                n166 = call "Convert to Dynamic Data8"("Array"=w335) -> ("Dynamic Data Type"=w339:dynamicdata)  [unwired: 3 in]
                n167 = Bundle By Name("dt"=w343, "Y"=w336) -> (w341:waveform(dbl))  [unwired: 1 in]
                n168 = Bundle By Name("dt"=w343, "Y"=w335) -> (w340:waveform(dbl))  [unwired: 1 in]
                n169 = property on="Linescan x voltages per scan point" class="WFGraph (strict)"("Value"=w336) -> ()  [unwired: 2 in, 2 out]
                n170 = property on="Linescan y voltages per scan point" class="WFGraph (strict)"("Value"=w335) -> ()  [unwired: 2 in, 2 out]
                n171 = property on="Linescan x waveform" class="WFGraph (strict)"("Value"=w341) -> ()  [unwired: 2 in, 2 out]
                n172 = Build Array(w341, w340) -> (w342:waveform(dbl)[])
                n173 = property on="Linescan y waveform" class="WFGraph (strict)"("Value"=w340) -> ()  [unwired: 2 in, 2 out]
                n174 = call "Build XY Graph4"("Y Input"=w339, "X Input"=w338) -> ("XY Graph"=w337:cluster{"Y":dbl[], "Y":dbl[]}[])  [unwired: 3 in, 6 out]
                n175 = property on="Final linescan xy voltage plot" class="XYGraph (strict)"("Value"=w337) -> ()  [unwired: 2 in, 2 out]
                n176 = call "GFG_core.vi"("Variable Name in"="linescan.xy.waveform", "Variant in"=w342, "Action"=enum16{"Init", "Set", "Get"}."Set") -> ()  [unwired: 10 in, 7 out]
              }
              frame True {
              }
            }
          }
          frame "FOCUS" {
            n177 = Variant To Data(type=TRUE, Variant=w389) -> (data=w381:bool)  [unwired: 1 in, 1 out]
            n178 = feedback #6(FALSE) -> (w384:bool)
            n179 = feedback-in #6(w381) -> ()
            n180 = Greater?(x=w381, y=w384) -> (0:w382:bool)
            n181 = case shown="False" w382 {
              tunnel: w380 -> [_ w409]
              tunnel: w379 -> [w403 _]
              tunnel: w378 -> [w402 _]
              frame False {
                w397 = scan_mode_main_settings_tab."2D line scan" ("scan mode main settings")
                n182 = call-poly "GFGpolyGet.vi"("Variable Name in"="MacroZipPath") -> ("Path"=w391:path)  [unwired: 8 in, 2 out]
                n183 = Equal? "No macro running?"(x=path "", y=w391) -> (x = y?=w390:bool)
                n184 = call "GFG_core.vi"("Variable Name in"="scan.mode.main.settings", "Action"=enum16{"Init", "Set", "Get", "Clear"}."Get") -> ("Variant Out"=w400:variant, "error out"=w401:errorcluster)  [unwired: 11 in, 5 out]
                n185 = Variant To Data(error in=w401, type=w397, Variant=w400) -> (data=w396:T9)  [unwired: 1 out]
                n186 = Equal?(x=w397, y=w396) -> (x = y?=w395:bool)
                n187 = And(x=w390, y=w395) -> (x .and. y?=w394:bool)
                n188 = case "Linescan active and no macro running?" shown="True" w394 {
                  tunnel: w403 -> [_ w405]
                  tunnel: w402 -> [_ w404]
                  frame False {
                  }
                  frame True {
                    n189 = Empty Array?(array=w405) -> (empty?=w406:bool)
                    n190 = case "Switch back to framescan (not instantly, only when display gets updated, so it keeps the last linescan frame until then)" shown="False" w406 {
                      tunnel: w405 -> [w408 _]
                      tunnel: w404 -> [w407 _]
                      frame False {
                        n191 = call "Recover_last_framescan_on_linescan_display.vi"("Time stamp of last confirm"=w407, "Last framescan image (updates when pressing \"Confirm\")"=w408) -> ()  [unwired: 9 in, 1 out]
                      }
                      frame True {
                      }
                    }
                  }
                }
              }
              frame True {
                # "Reset ROI, when FOCUS"
                n192 = call-poly "GFGpolyGet.vi"() -> ("Image Refs Out"=w416:T12)  [unwired: 10 in, 1 out]
                n193 = Cluster To Array(cluster=w416) -> (array=w414:T11[])
                n194 = Index Array(array=w414, index=10) -> (element=w413:T11)
                n195 = property class="ImageControl"(reference=w409, "Value"=w413) -> (reference out=w411:refnum<vi>, error out=w410:errorcluster)  [unwired: 1 in]
                n196 = property class="ImageControl"(reference=w411, error in=w410, "ROI"=T3 {"Global Rectangle"=[], "Contours"=[]}) -> ()  [unwired: 2 out]
              }
            }
          }
          frame "Record" {
            n197 = Variant To Data(type=TRUE, Variant=w423) -> (data=w424:bool)  [unwired: 1 in, 1 out]
            n198 = feedback #7(FALSE) -> (w427:bool)
            n199 = feedback-in #7(w424) -> ()
            n200 = Greater?(x=w424, y=w427) -> (0:w425:bool)
            n201 = case shown="True" w425 {
              tunnel: w422 -> [_ w429]
              frame False {
              }
              frame True {
                # "Reset ROI, when Record"
                n202 = property class="ImageControl"(reference=w429, "ROI"=T3 {"Global Rectangle"=[], "Contours"=[]}) -> ()  [unwired: 1 in, 2 out]
              }
            }
          }
          frame "QUIT" {
            n203 = Variant To Data(type=TRUE, Variant=w437) -> (data=w436:bool)  [unwired: 1 in, 1 out]
          }
        }
      }
    }
  }
